vi "Code 1 - Pre-processing.vi"() -> ()   [LabVIEW 2020]
panel:
  out "Data":dbl[][](array[numeric])
  out "size(s)":i32[](array[numeric])
  out "Data OUT":dbl[][](array[numeric])
  out "transposed array 2":dbl[][](array[numeric])
  out "Muscle organized":dbl[][](array[numeric])
  out "Demographics":dbl[][](array[numeric])
  out "Motor score organized":dbl[][](array[numeric])
  in  "Number of participants":dbl
  out "Acute I, Acute II, \nAcute 3, Chronic":dbl[][](array[numeric])
  out "Array":dbl[][](array[numeric])
  out "transposed array":dbl[][](array[numeric])
  out "data":string
  out "new file path":path
  # "Columns"
  # "Participant code Code\nAge (years)\nGender (1_M, 2_F)\nTime post-SCI (months)\nASIA  (1_A, 2_B, 3_C, 4_D)\nLevel of injury\nGroup (1_Control , 2_FES-T)\nTime (0-bas, 1- 8wk, 2- 6mo)\n(R) Anterior Deltoid\n(R) Elbow Flexors\n(R) Elbow Extensors\n(R) Wrist Extensors\n(R) Extensor Digitorum (DIII)\n(R) Opponens Pollicis\n(R) Flexor Pollicis Longus\n(R) Finger Flexors (DIII)\n(R) Finger Abductors\n(R) First Dorsal Interossei\n(R) Total (out of 50)\n(L) Anterior Deltoid\n(L) Elbow Flexors\n(L) Elbow Extensors\n(L) Wrist Extensors\n(L) Extensor Digitorum (DIII)\n(L) Opponens Pollicis\n(L) Flexor Pollicis Longus\n(L) Finger Flexors (DIII)\n(L) Finger Abductors\n(L) First Dorsal Interossei\n(L) Total (out of 50)"
  # "0\n1\n2\n3\n4\n5\n6\n7\n8\n9\n10\n11\n12\n13\n14\n15\n16\n17\n18\n19\n20\n21\n22\n23\n24\n25\n26\n27\n28\n29"
  # "Column"
  # "0\n1\n2\n3\n4\n5\n6\n7\n8\n9"
  # "Patientennummer\nSex\nAgeAtDOI\nCause\nExamStage\nAIS\nRML\nLML\nCOMPL\nRMS_C5\nRMS_C6\nRMS_C7\nRMS_C8\nRMS_T1\nRMS_L2\nRMS_L3\nRMS_L4\nRMS_L5\nRMS_S1\nLMS_C5\nLMS_C6\nLMS_C7\nLMS_C8\nLMS_T1\nLMS_L2\nLMS_L3\nLMS_L4\nLMS_L5\nLMS_S1"
  # "0\n1\n2\n3\n4\n5\n6\n7\n8\n9\n10\n11\n12\n13\n14\n15\n16\n17\n18\n19"
  # "Rows at the last column"
  # "Columns"
  # "Participant code Code\nAge (years)\nGender (1_M, 2_F)\nTime post-SCI (months)\nASIA  (1_A, 2_B, 3_C, 4_D)\nLevel of injury\nGroup (1_Control , 2_FES-T)\nTime (0-bas, 1- 8wk, 2- 6mo)\n(R) Anterior Deltoid\n(R) Elbow Flexors\n(R) Elbow Extensors\n(R) Wrist Extensors\n(R) Extensor Digitorum (DIII)\n(R) Opponens Pollicis\n(R) Flexor Pollicis Longus\n(R) Finger Flexors (DIII)\n(R) Finger Abductors\n(R) First Dorsal Interossei\n(R) Total (out of 50)\n(L) Anterior Deltoid\n(L) Elbow Flexors\n(L) Elbow Extensors\n(L) Wrist Extensors\n(L) Extensor Digitorum (DIII)\n(L) Opponens Pollicis\n(L) Flexor Pollicis Longus\n(L) Finger Flexors (DIII)\n(L) Finger Abductors\n(L) First Dorsal Interossei\n(L) Total (out of 50)"
  # "0\n1\n2\n3\n4\n5\n6\n7\n8\n9\n10\n11\n12\n13\n14\n15\n16\n17\n18\n19\n20\n21\n22\n23\n24\n25\n26\n27\n28\n29"
  # "NEW"
  # "0\n1\n2\n3\n4\n5\n6\n7\n8\n9\n10\n11\n12\n13\n14\n15\n16\n17\n18\n19\n20\n21\n22\n23\n24\n25\n26"
  # "Patientennummer\nSex\nAgeAtDOI\nCause\nExamStage\nAIS\nNLI\nRMS_C5\nRMS_C6\nRMS_C7\nRMS_C8\nRMS_T1\nRMS_L2\nRMS_L3\nRMS_L4\nRMS_L5\nRMS_S1\nLMS_C5\nLMS_C6\nLMS_C7\nLMS_C8\nLMS_T1\nLMS_L2\nLMS_L3\nLMS_L4\nLMS_L5\nLMS_S1"
  # "748 SCI with complete data\n51 excluded (missing data)"
  # "2\t1\t0\t0\t0\t1\t2\t1\t1\t2\t2\t0\t0\t0\t0\t0\t1\t0\t0\t0\n3\t3\t2\t1\t1\t3\t3\t3\t2\t1\t3\t2\t2\t1\t0\t2\t3\t2\t1\t1\n3\t3\t3\t2\t1\t3\t3\t3\t3\t3\t3\t2\t2\t1\t0\t2\t3\t2\t2\t2\n3\t3\t3\t2\t1\t3\t3\t3\t3\t3\t3\t2\t2\t1\t0\t2\t3\t3\t2\t2"
  # "Columns"
  # "Participant code Code\nAge (years)\nGender (1_M, 2_F)\nTime post-SCI (months)\nASIA  (1_A, 2_B, 3_C, 4_D)\nLevel of injury\nGroup (1_Control , 2_FES-T)\nTime (0-bas, 1- 8wk, 2- 6mo)\n(R) Anterior Deltoid\n(R) Elbow Flexors\n(R) Elbow Extensors\n(R) Wrist Extensors\n(R) Extensor Digitorum (DIII)\n(R) Opponens Pollicis\n(R) Flexor Pollicis Longus\n(R) Finger Flexors (DIII)\n(R) Finger Abductors\n(R) First Dorsal Interossei\n(R) Total (out of 50)\n(L) Anterior Deltoid\n(L) Elbow Flexors\n(L) Elbow Extensors\n(L) Wrist Extensors\n(L) Extensor Digitorum (DIII)\n(L) Opponens Pollicis\n(L) Flexor Pollicis Longus\n(L) Finger Flexors (DIII)\n(L) Finger Abductors\n(L) First Dorsal Interossei\n(L) Total (out of 50)"
  # "0\n1\n2\n3\n4\n5\n6\n7\n8\n9\n10\n11\n12\n13\n14\n15\n16\n17\n18\n19\n20\n21\n22\n23\n24\n25\n26\n27\n28\n29"
  # "NEW"
  # "0\n1\n2\n3\n4\n5\n6\n7\n8\n9\n10\n11\n12\n13\n14\n15\n16\n17\n18\n19\n20\n21\n22\n23\n24\n25\n26"
  # "Patientennummer\nSex\nAgeAtDOI\nCause\nExamStage\nAIS\nNLI\nRMS_C5\nRMS_C6\nRMS_C7\nRMS_C8\nRMS_T1\nRMS_L2\nRMS_L3\nRMS_L4\nRMS_L5\nRMS_S1\nLMS_C5\nLMS_C6\nLMS_C7\nLMS_C8\nLMS_T1\nLMS_L2\nLMS_L3\nLMS_L4\nLMS_L5\nLMS_S1"
  # "NEW"
  # "0\n1\n2\n3\n4\n5\n6\n7\n8\n9\n10\n11\n12\n13\n14\n15\n16\n17\n18\n19\n20\n21\n22\n23\n24\n25\n26"
  # "Patientennummer\nSex\nAgeAtDOI\nCause\nExamStage\nAIS\nNLI\nRMS_C5\nRMS_C6\nRMS_C7\nRMS_C8\nRMS_T1\nRMS_L2\nRMS_L3\nRMS_L4\nRMS_L5\nRMS_S1\nLMS_C5\nLMS_C6\nLMS_C7\nLMS_C8\nLMS_T1\nLMS_L2\nLMS_L3\nLMS_L4\nLMS_L5\nLMS_S1"
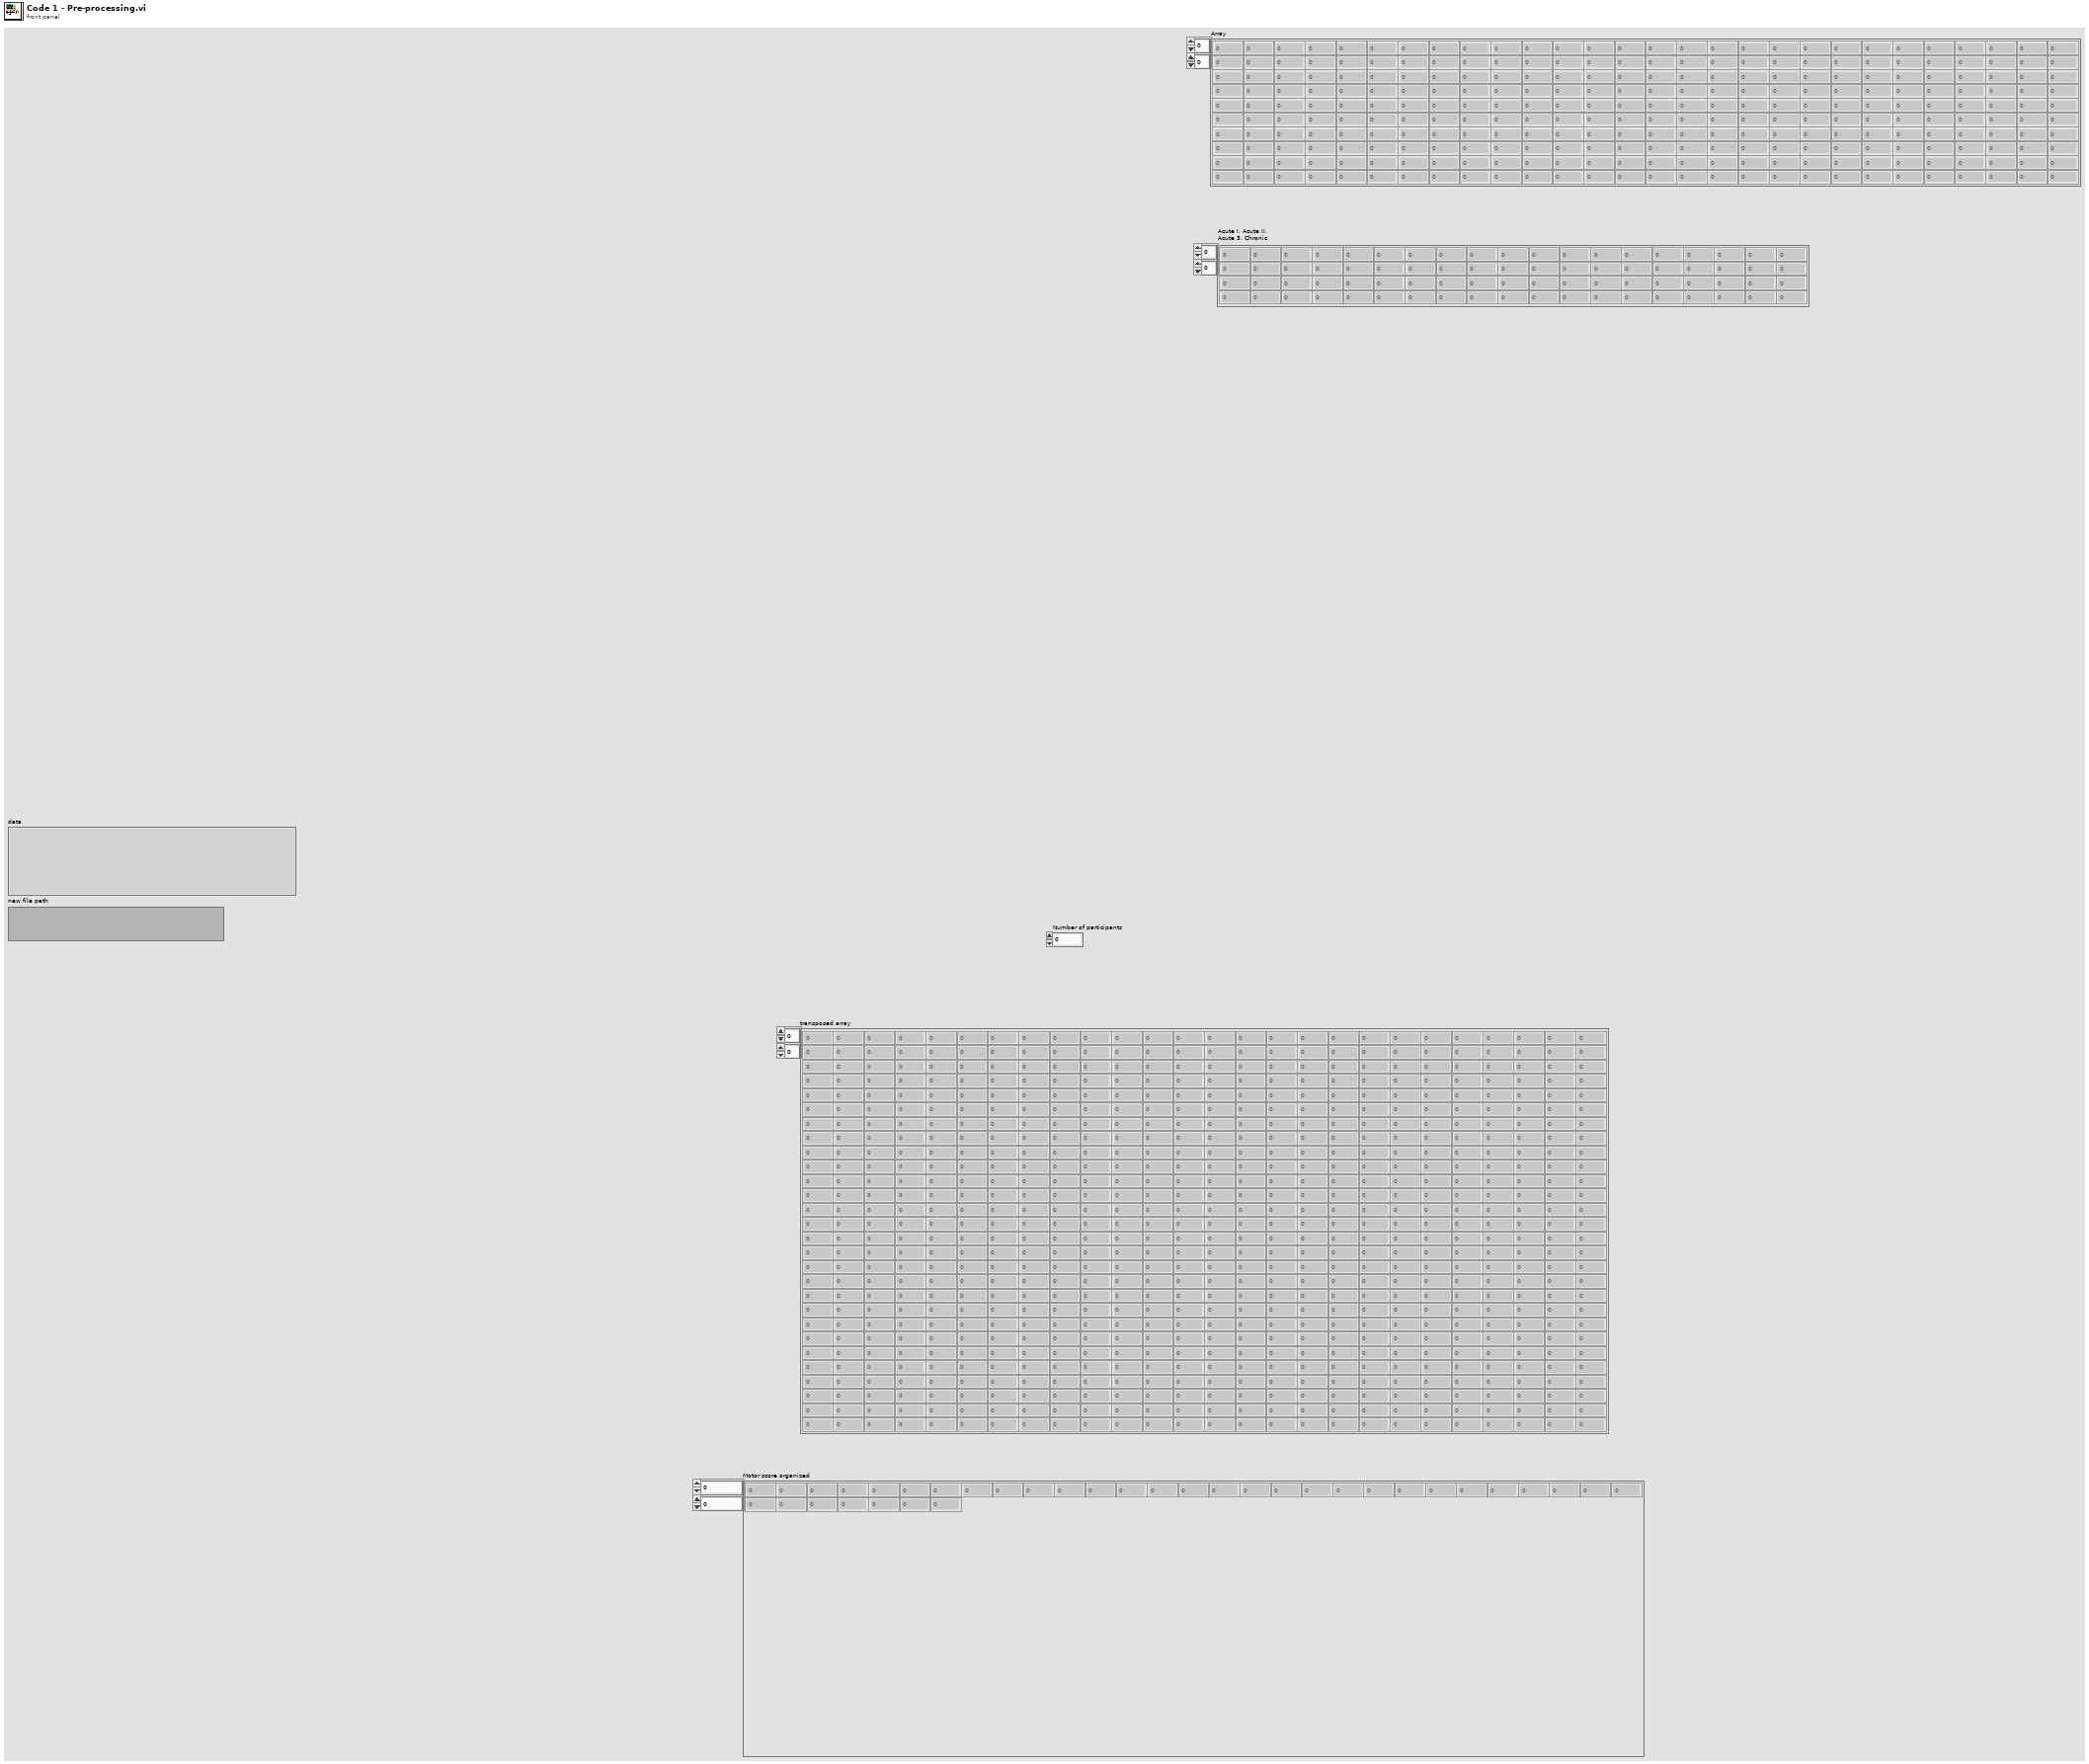
[diagram p1: front panel]
types:
  T1 = enum16{"open", "open or create", "create or replace", "create", "open (read only)"}
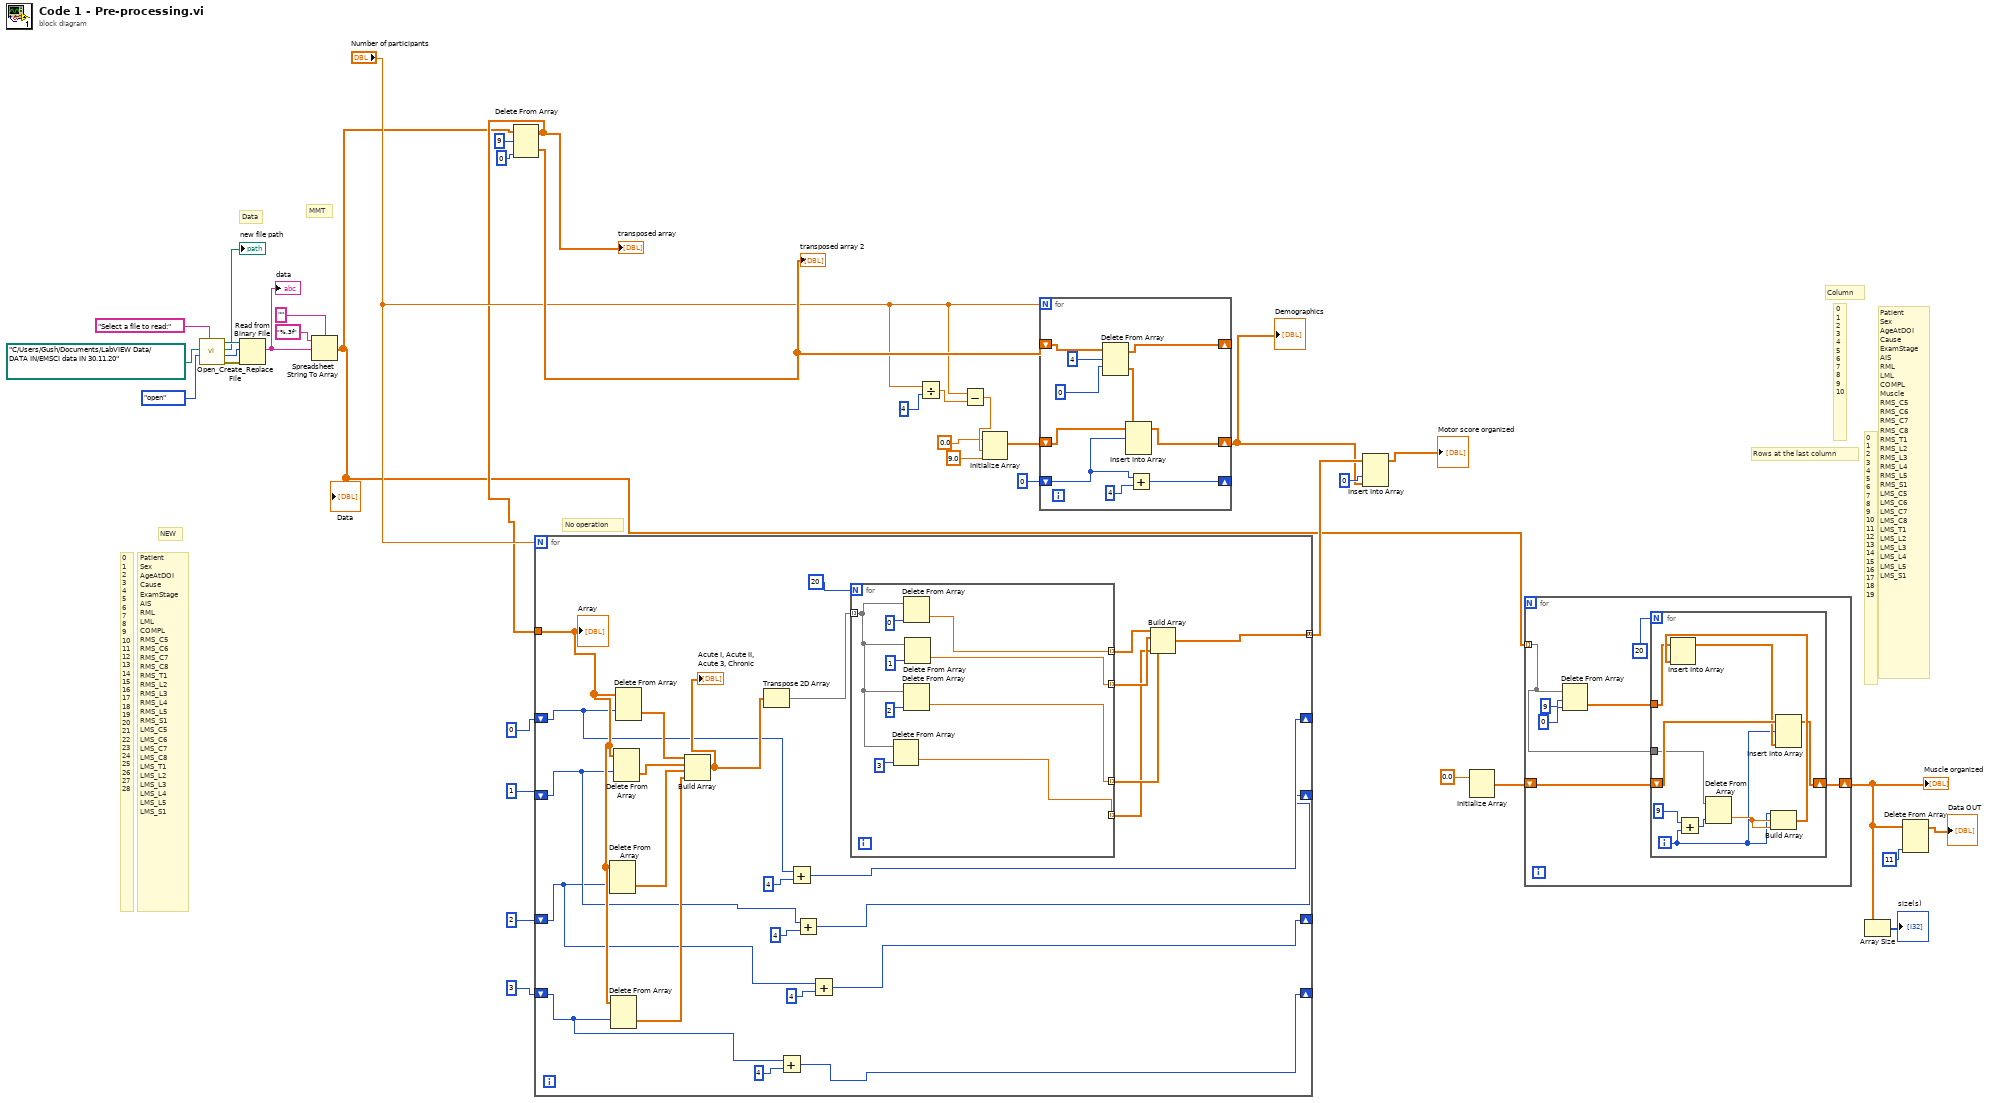
[diagram p0: block diagram]
diagram:
  # "Patient\nSex\nAgeAtDOI\nCause\nExamStage\nAIS\nRML\nLML\nCOMPL\nMuscle\nRMS_C5\nRMS_C6\nRMS_C7\nRMS_C8\nRMS_T1\nRMS_L2\nRMS_L3\nRMS_L4\nRMS_L5\nRMS_S1\nLMS_C5\nLMS_C6\nLMS_C7\nLMS_C8\nLMS_T1\nLMS_L2\nLMS_L3\nLMS_L4\nLMS_L5\nLMS_S1"
  # "Rows at the last column"
  # "Column"
  # "0\n1\n2\n3\n4\n5\n6\n7\n8\n9\n10\n11\n12\n13\n14\n15\n16\n17\n18\n19"
  # "0\n1\n2\n3\n4\n5\n6\n7\n8\n9\n10"
  # "No operation"
  # "NEW"
  # "Patient\nSex\nAgeAtDOI\nCause\nExamStage\nAIS\nRML\nLML\nCOMPL\nRMS_C5\nRMS_C6\nRMS_C7\nRMS_C8\nRMS_T1\nRMS_L2\nRMS_L3\nRMS_L4\nRMS_L5\nRMS_S1\nLMS_C5\nLMS_C6\nLMS_C7\nLMS_C8\nLMS_T1\nLMS_L2\nLMS_L3\nLMS_L4\nLMS_L5\nLMS_S1"
  # "0\n1\n2\n3\n4\n5\n6\n7\n8\n9\n10\n11\n12\n13\n14\n15\n16\n17\n18\n19\n20\n21\n22\n23\n24\n25\n26\n27\n28"
  # "MMT"
  # "Data"
  n1 = call <vilib>:"Open_Create_Replace File.vi"("prompt"="Select a file to read:", "function (open:0)"=T1."open", "start path  (Not A Path)"=path "C:/Users/Gush/Documents/LabVIEW Data/DATA IN/EMSCI data IN 30.11.20") -> ("error out"=w31:errorcluster, "file size (bytes)"=w36:i32, "new file path"=→"new file path":path, "refnum"=w35:refnum<file>)  [unwired: 5 in]
  n2 = Read from Binary File ("Read File")(8:w31, 10:w36, 11:w35) -> (2:w28:string)  [unwired: 3 in, 3 out]
  "data" <- w28
  n3 = Spreadsheet String To Array(delimiter (Tab)="", format string="%.3f" ("String"), spreadsheet string=w28) -> (array=w1:dbl[][])  [unwired: 1 in]
  "Data" <- w1
  n4 = Delete From Array(array=w1, length=9, index (col)=0) -> (deleted portion=w17:dbl[][], array with subset deleted=w4:dbl[][])  [unwired: 1 in]
  "transposed array" <- w4
  "transposed array 2" <- w17
  n5 = for {
    N: "Number of participants" -> [_]
    tunnel: w4 -> [w53]
    shift-right: [w42] -> _
    shift-left: 2 -> [w43]
    tunnel: [w58] -> w18 mode=concatenating
    shift-right: [w48] -> _
    shift-left: 0 -> [w49]
    shift-right: [w45] -> _
    shift-left: 1 -> [w46]
    shift-right: [w39] -> _
    shift-left: 3 -> [w40]
    n6 = Delete From Array(array=w53, index (row)=w43) -> (deleted portion=w55:dbl[])  [unwired: 2 in, 1 out]
    n7 = Delete From Array(array=w53, index (row)=w40) -> (deleted portion=w52:dbl[])  [unwired: 2 in, 1 out]
    n8 = Delete From Array(array=w53, index (row)=w46) -> (deleted portion=w56:dbl[])  [unwired: 2 in, 1 out]
    n9 = Delete From Array(array=w53, index (row)=w49) -> (deleted portion=w57:dbl[])  [unwired: 2 in, 1 out]
    n10 = Build Array(w57, w56, w55, w52) -> (w54:dbl[][])
    "Acute I, Acute II, \nAcute 3, Chronic" <- w54
    n11 = Transpose 2D Array(2D array=w54) -> (transposed array=w62:dbl[][])
    n12 = Add(x=w40, y=4) -> (x+y=w39:i32)
    n13 = Add(x=w49, y=4) -> (x+y=w48:i32)
    n14 = Add(x=w46, y=4) -> (x+y=w45:i32)
    n15 = Add(x=w43, y=4) -> (x+y=w42:i32)
    n16 = for {
      N: 20 -> [_]
      tunnel: w62 -> [w67] mode=indexing
      tunnel: [w66] -> w60 mode=indexing
      tunnel: [w65] -> w59 mode=indexing
      tunnel: [w64] -> w51 mode=indexing
      tunnel: [w63] -> w38 mode=indexing
      n17 = Delete From Array(array=w67, index=3) -> (deleted portion=w63:dbl)  [unwired: 1 in, 1 out]
      n18 = Delete From Array(array=w67, index=0) -> (deleted portion=w66:dbl)  [unwired: 1 in, 1 out]
      n19 = Delete From Array(array=w67, index=2) -> (deleted portion=w64:dbl)  [unwired: 1 in, 1 out]
      n20 = Delete From Array(array=w67, index=1) -> (deleted portion=w65:dbl)  [unwired: 1 in, 1 out]
    }
    n21 = Build Array(w60, w59, w51, w38) -> (w58:dbl[][])
    "Array" <- w53
  }
  n22 = Divide(x="Number of participants", y=4) -> (x/y=w15:dbl)
  n23 = Subtract(x="Number of participants", y=w15) -> (x-y=w14:dbl)
  n24 = Initialize Array(0.0, w14, 9.0) -> (w13:dbl[][])
  n25 = for {
    N: "Number of participants" -> [_]
    shift-right: [w79] -> _
    shift-left: w17 -> [w81]
    shift-right: [w73] -> w10
    shift-left: w13 -> [w78]
    shift-right: [w74] -> _
    shift-left: 0 -> [w76]
    n26 = Delete From Array(array=w81, length=4, index (row)=0) -> (deleted portion=w77:dbl[][], array with subset deleted=w79:dbl[][])  [unwired: 1 in]
    n27 = Insert Into Array(array=w78, index (row)=w76, new element=w77) -> (w73:dbl[][])  [unwired: 1 in]
    n28 = Add(x=w76, y=4) -> (x+y=w74:i32)
  }
  "Demographics" <- w10
  n29 = Insert Into Array(array=w18, index (col)=0, new element=w10) -> (→"Motor score organized":dbl[][])  [unwired: 1 in]
  n30 = Initialize Array(0.0) -> (w23:dbl[][])  [unwired: 2 in]
  n31 = for {
    tunnel: w1 -> [w82] mode=indexing
    shift-right: [w83] -> w2
    shift-left: w23 -> [w85]
    n32 = Delete From Array(array=w82, length=9, index=0) -> (deleted portion=w86:dbl[])  [unwired: 1 out]
    n33 = for {
      N: 20 -> [_]
      tunnel: w86 -> [w93]
      shift-right: [w90] -> w83
      shift-left: w85 -> [w98]
      tunnel: w82 -> [w96]
      i -> [w89]
      n34 = Add(x=9, y=w89) -> (x+y=w97:i32)
      n35 = Delete From Array(array=w96, index=w97) -> (deleted portion=w95:dbl)  [unwired: 1 in, 1 out]
      n36 = Build Array(w89, w95, w95) -> (w94:dbl[])
      n37 = Insert Into Array(array=w93, new element=w94) -> (w92:dbl[])  [unwired: 1 in]
      n38 = Insert Into Array(array=w98, index (row)=w89, new element=w92) -> (w90:dbl[][])  [unwired: 1 in]
    }
  }
  "Muscle organized" <- w2
  n39 = Array Size(array=w2) -> (size(s)=→"size(s)":i32[])
  n40 = Delete From Array(array=w2, index (col)=11) -> (array with subset deleted=→"Data OUT":dbl[][])  [unwired: 2 in, 1 out]
